vi "Data Latch Slave.vi"(3 "Done Sending":bool, 4 "[S]":T1, 5 "Done Reading":bool, 6 "[S]`":T1) -> (0 "Send Message":bool, 1 "Read Message":bool, 2 "[S] out":T1)   [LabVIEW 2010]
uses:
  Data Latch.ctl
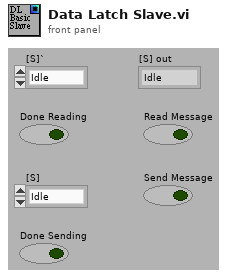
[diagram p1: front panel]
types:
  T1 = typedef "Data Latch.ctl" = enum8{"Idle", "Sending", "Sent", "Receiving", "Received"}
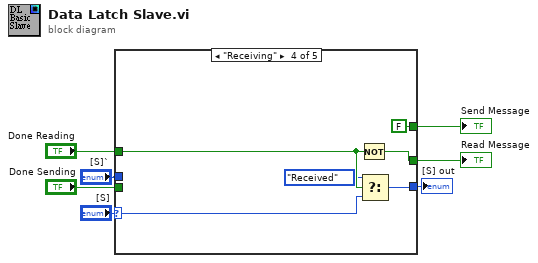
[diagram p0: block diagram]
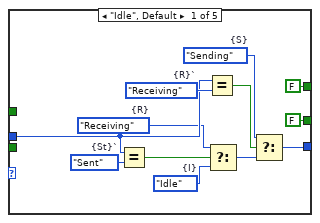
[diagram p2: hidden frame]
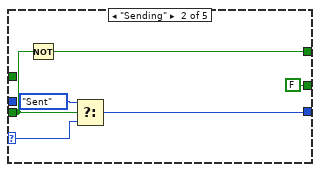
[diagram p3: hidden frame]
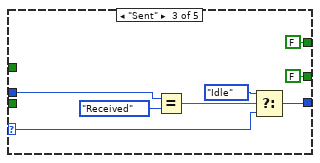
[diagram p4: hidden frame]
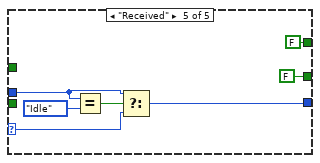
[diagram p5: hidden frame]
diagram:
  n1 = case shown="\"Receiving\"" "[S]" {
    selector: "[S]" -> [_ w24 w28 w36 w43]
    tunnel: "[S]`" -> [w17 _ w32 _ w42]
    tunnel: [w10 w20 w26 w35 w41] -> w3
    tunnel: "Done Reading" -> [_ _ _ w37 _]
    tunnel: [FALSE FALSE FALSE w38 FALSE] -> w5
    tunnel: [FALSE w21 FALSE FALSE FALSE] -> w6
    tunnel: "Done Sending" -> [_ w22 _ _ _]
    frame "Idle", Default {
      w11 = Data_Latch."Idle"  # {I}
      w15 = Data_Latch."Sending"  # {S}
      w13 = Data_Latch."Receiving"  # {R}
      w18 = Data_Latch."Receiving"  # {R}`
      w19 = Data_Latch."Sent"  # {St}`
      n2 = Equal?(x=w17, y=w19) -> (x = y?=w14:bool)
      n3 = Equal?(x=w17, y=w18) -> (x = y?=w16:bool)
      n4 = Select(t=w13, s=w14, f=w11) -> (s? t:f=w12:T1)
      n5 = Select(t=w15, s=w16, f=w12) -> (s? t:f=w10:T1)
    }
    frame "Sending" {
      n6 = Not(x=w22) -> (.not. x?=w21:bool)
      n7 = Select(t=Data_Latch."Sent", s=w22, f=w24) -> (s? t:f=w20:T1)
    }
    frame "Sent" {
      n8 = Equal?(x=w32, y=Data_Latch."Received") -> (x = y?=w29:bool)
      n9 = Select(t=Data_Latch."Idle", s=w29, f=w28) -> (s? t:f=w26:T1)
    }
    frame "Receiving" {
      n10 = Not(x=w37) -> (.not. x?=w38:bool)
      n11 = Select(t=Data_Latch."Received", s=w37, f=w36) -> (s? t:f=w35:T1)
    }
    frame "Received" {
      n12 = Equal?(x=w42, y=Data_Latch."Idle") -> (x = y?=w44:bool)
      n13 = Select(t=w42, s=w44, f=w43) -> (s? t:f=w41:T1)
    }
  }
  "Send Message" <- w6
  "Read Message" <- w5
  "[S] out" <- w3
